vi "Update_xPos.vi"(7 "NumOfAxis":i32, 8 "error in (no error)":errorcluster, 11 "VISA resource name":refnum<visa-resource-name>) -> (0 "error out":errorcluster, 1 "x_Moving":bool, 2 "Position":dbl[](array[numeric]), 3 "tickcount_pos":u32)   [LabVIEW 2013, in "Micos_uic.lvlib"]
doc: "Performs an instrument error query before terminating the software connection to the instrument."
uses:
  <instrlib>/Micos_uic/Micos_uic.lvlib
  <vilib>/Utility/error.llb/DialogType.ctl
  <instrlib>/Micos_uic/Public/Position_Micos.vi
  <vilib>/regexp/Match Regular Expression.xnode
panel:
  out "Read Buffer":string
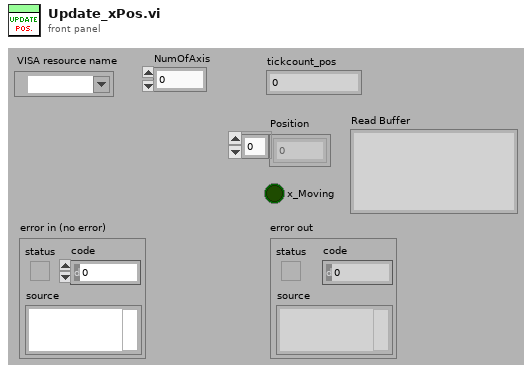
[diagram p1: front panel]
types:
  T1 = typedef "DialogType.ctl" = u16
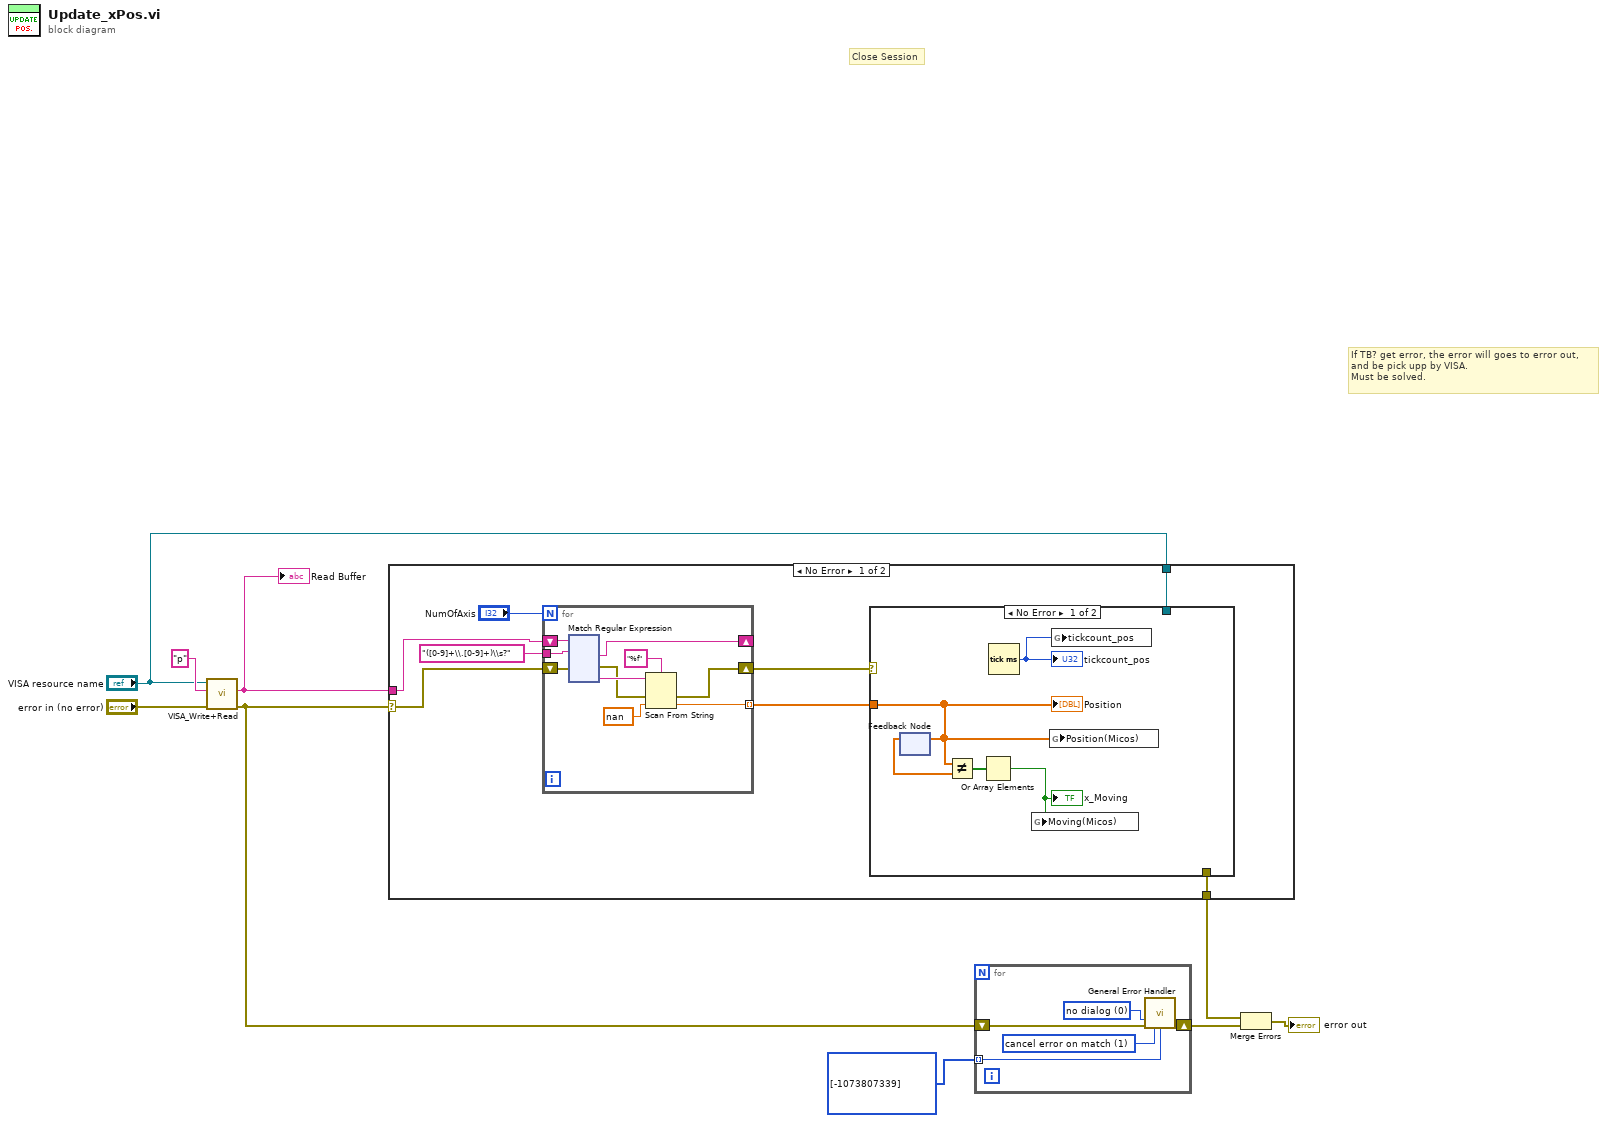
[diagram p0: block diagram]
diagram:
  # "If TB? get error, the error will goes to error out, \nand be pick upp by VISA.\nMust be solved."
  # "Close Session"
  n1 = call <instrlib>:"VISA_Write+Read.vi"("error in (no error)"="error in (no error)", "Write Buffer"="p" ("string"), "VISA resource name"="VISA resource name") -> ("error out"=w1:errorcluster, "readout"=w7:string)  [unwired: 6 in, 1 out]
  "Read Buffer" <- w7
  n2 = case shown="No Error" w1 {
    selector: w1 -> [w12 w147]
    tunnel: w7 -> [w15 _]
    tunnel: "VISA resource name" -> [w11 _]
    tunnel: [w10 w147] -> w2
    frame No Error {
      n3 = for {
        N: "NumOfAxis" -> [_]
        shift-right: [w32] -> _
        shift-left: w15 -> [w33]
        tunnel: "([0-9]+\\.[0-9]+)\\s?" ("regular expression") -> [w31]
        tunnel: [w29] -> w14 mode=indexing
        shift-right: [w27] -> w13
        shift-left: w12 -> [w25]
        n4 = xnode "Match Regular Expression"("input string"=w33, "regular expression"=w31, "error in"=w25) -> ("after match"=w32:string, "error out"=w26:errorcluster, "submatch 1"=w30:string)  [unwired: 3 in, 3 out]
        n5 = Scan From String(format string="%f", input string=w30, error in=w26, default 1=nan ("default value 1")) -> (error out=w27:errorcluster, output 1=w29:dbl)  [unwired: 1 in, 2 out]
      }
      n6 = case shown="No Error" w13 {
        selector: w13 -> [_ w23]
        tunnel: w14 -> [w21 _]
        tunnel: w11 -> [_ _]
        tunnel: [_ w23] -> w10
        frame No Error {
          n7 = feedback #1() -> (w19:dbl[])  [unwired: 1 in]
          n8 = feedback-in #1(w21) -> ()
          n9 = Not Equal?(x=w21, y=w19) -> (x != y?=w20:bool[])
          n10 = Or Array Elements(Boolean array=w20) -> (logical OR=w18:bool)
          "x_Moving" <- w18
          n11 = Tick Count (ms)() -> (millisecond timer value=w22:u32)
          "tickcount_pos" <- w22
          n12 = global write "Position_Micos.vi" "Moving(Micos)"(w18) -> ()
          n13 = global write "Position_Micos.vi" "Position(Micos)"(w21) -> ()
          n14 = global write "Position_Micos.vi" "tickcount_pos"(w22) -> ()
          "Position" <- w21
        }
        frame Error {
          # "removed visa clear ??"
        }
      }
    }
    frame Error {
    }
  }
  n15 = for {
    tunnel: i32[] [-1073807339] -> [w148] mode=indexing
    shift-right: [w152] -> w4
    shift-left: w1 -> [w150]
    w149 = T1 0 items=["no dialog", "OK message", "continue or stop message", "OK message + warnings", "continue/stop + warnings"] ("type of dialog (OK msg:1)")
    w151 = 1 items=["no exception", "cancel error on match", "set error on match"] ("[exception action] (none:0)")
    n16 = call <vilib>:"General Error Handler.vi"("type of dialog (OK msg:1)"=w149, "error in (no error)"=w150, "[exception action] (none:0)"=w151, "[exception code]"=w148) -> ("error out"=w152:errorcluster)  [unwired: 7 in, 4 out]
  }
  n17 = Merge Errors(w2, w4) -> (→"error out":errorcluster)
